vi "Set JSON CFG.vi"(10 "<JSON>Data SInk CFG":string, 11 "TDMS Sink in":refnum<class "TDMS Sink.lvclass">) -> (3 "TDMS Sink out":refnum<class "TDMS Sink.lvclass">)   [LabVIEW 2024, in "TDMS Sink.lvclass"]
uses:
  TDMS Sink.lvclass
  TDMS Sink.lvclass/TDMS Sink.ctl
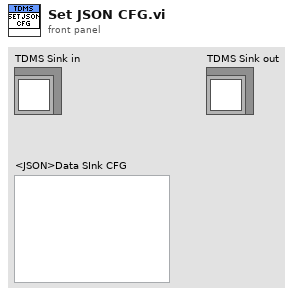
[diagram p1: front panel]
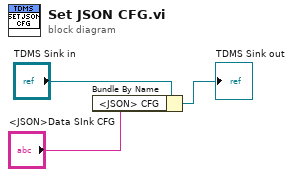
[diagram p0: block diagram]
diagram:
  n1 = Bundle By Name(cluster="TDMS Sink in", "<JSON> CFG"="<JSON>Data SInk CFG") -> (→"TDMS Sink out":refnum<class "TDMS Sink.lvclass">)
